vi "2D_array_statistics.vi"(4 "N Sig hist range":dbl=5.0 format="%.1f", 6 "Array":dbl[][](array[numeric])=array100x100[10000 elements] format="%.2f") -> (0 "1D array":dbl[](array[numeric]), 1 "mean 2":dbl=0.456875 format="%.2f", 2 "RMS 2":dbl=6.561297508877341 format="%.2f", 3 "median 3":dbl format="%.2f")   [LabVIEW 2017]
uses:
  <vilib>/Analysis/6fits.llb/Curve Fitting Criteria.ctl
  <vilib>/Analysis/5stat.llb/RMS (DBL).vi
  <vilib>/Analysis/baseanly.llb/Mean (DBL).vi
  <vilib>/Analysis/NI_AALBase.lvlib
  <vilib>/Analysis/NI_AALPro.lvlib
panel:
  out "RMS 2":dbl=6.561297508877341 format="%.2f"
  out "mean 2":dbl=0.456875 format="%.2f"
  out "median 2":dbl format="%.2f"
  out "Waveform Graph":dbl[](graph)
  in  "min":dbl=-45.47220756214139 format="%0.2f"
  in  "max":dbl=46.385957562141385 format="%0.2f"
  in  "# bins":i32=13
  out "# outside":cluster{"total":i32, "below":i32, "above":i32}={"total"=35, "below"=22, "above"=13}
  out "Histogram Graph":T1(graph)=[{"X Values"=[-41.93920121120744, -34.873188509339535, -27.80717580747163, -20.74116310560372, -13.675150403735815, -6.609137701867908, 0.4568749999999966, 7.5228877018679015, 14.588900403735806, 21.654913105603715, 28.720925807471623, 35.78693850933953, 42.85295121120743], "Histogram: h(x)"=[0, 0, 0, 17, 301, 1746, 3308, 2047, 414, 27, 1, 0, 0]}, {"X Values"=[-41.93920121120744, -34.873188509339535, -27.80717580747163, -20.74116310560372, -13.675150403735815, -6.609137701867908, 0.4568749999999966, 7.5228877018679015, 14.588900403735806, 21.654913105603715, 28.720925807471623, 35.78693850933953, 42.85295121120743], "Histogram: h(x)"=[16, 41, 106, 338, 911, 1746, 3317, 2047, 901, 377, 105, 44, 16]}]
  in  "method":T2=1 items=["Least Square", "Least Absolute Residual", "Bisquare"]
  out "Amplitude":dbl=3317.070983574361 format="%.2f"
  out "STDev":dbl=6.680329359755373 format="%.2f"
  out "Center":dbl=0.958994388159082 format="%.2f"
  out "auze 3":u32=10000
  out "auze 2":u32=2000
  out "auze":u32=8000
  out "size":u16[](array[numeric])=[100, 100]
  out "RMS":dbl=11.6418383428048 format="%.3g"
  out "mean":dbl=0.4562 format="%.3g"
  out "median":dbl format="%.3f"
  # "Least Absolute Residual"
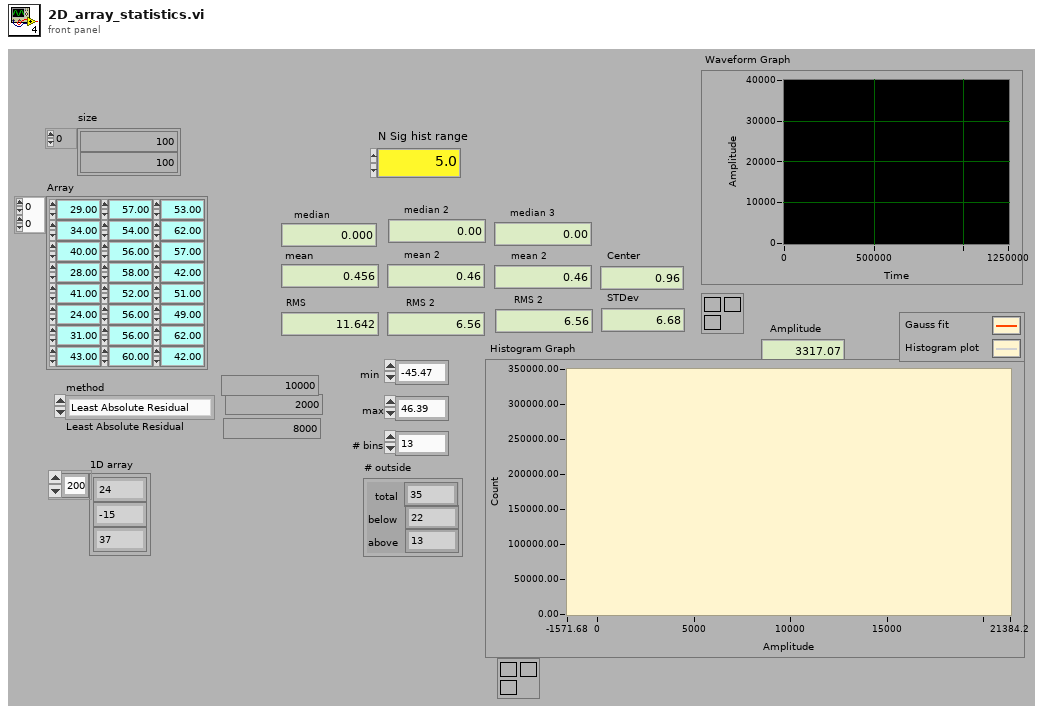
[diagram p1: front panel]
types:
  T1 = cluster{"X Values":dbl[], "Histogram: h(x)":i32[]}[]
  T2 = typedef "NI_AALPro.lvlib/Curve Fitting Criteria.ctl" = u16
  T3 = cluster{"X Values":dbl[], "Histogram: h(x)":i32[]}
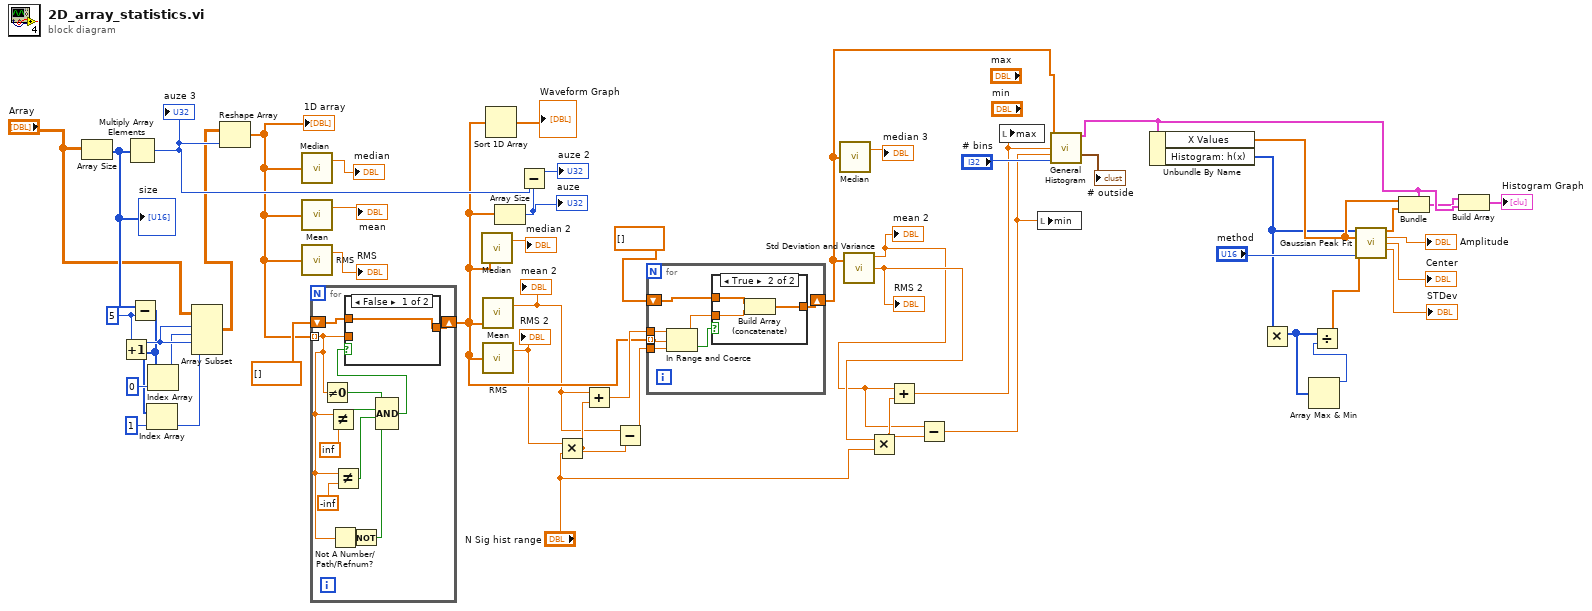
[diagram p0: block diagram]
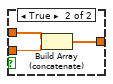
[diagram p3: hidden frame]
diagram:
  w29 = 5 ("y")
  n1 = Array Size(array="Array") -> (size(s)=w31:i32[])
  "size" <- w31
  n2 = Increment(x=w29) -> (x+1=w28:i32)
  n3 = Multiply Array Elements(1:w31) -> (0:w47:i32)
  "auze 3" <- w47
  n4 = Subtract(x=w31, y=w29) -> (x-y=w23:i32[])
  n5 = Index Array(array=w23, index=1) -> (element=w22:i32)
  n6 = Index Array(array=w23, index=0) -> (element=w25:i32)
  n7 = Array Subset(array="Array", index (row)=w28, length (row)=w25, index (col)=w28, length (col)=w22) -> (w24:dbl[][])
  n8 = Reshape Array(w24, w47) -> (w16:dbl[])
  "1D array" <- w16
  n9 = call <vilib>:"Median.vi"("X"=w16) -> ("median"=→"median":dbl)  [unwired: 1 out]
  n10 = call-poly <vilib>:"Mean.vi"("X"=w16) -> ("mean"=→"mean":dbl)  [unwired: 1 out]
  n11 = call-poly <vilib>:"RMS.vi"("X"=w16) -> ("rms value"=→"RMS":dbl)  [unwired: 1 out]
  n12 = for {
    tunnel: w16 -> [w53] mode=indexing
    shift-right: [w60] -> w7
    shift-left: dbl[] [] -> [w61]
    n13 = Not Equal To 0?(x=w53) -> (x != 0?=w57:bool)
    n14 = Not Equal?(x=w53, y=inf) -> (x != y?=w56:bool)
    n15 = Not A Number/Path/Refnum?(number/path/refnum=w53) -> (NaN/Path/Refnum?=w52:bool)
    n16 = Not Equal?(x=w53, y=-inf) -> (x != y?=w55:bool)
    n17 = Not(x=w52) -> (.not. x?=w51:bool)
    n18 = Compound Arithmetic op=AND(w57, w56, w55, w51) -> (w58:bool)
    n19 = case shown="False" w58 {
      tunnel: w53 -> [_ w65]
      tunnel: w61 -> [w62 w64]
      tunnel: [w62 w63] -> w60
      frame False {
      }
      frame True {
        n20 = Build Array (concatenate)(w64, w65) -> (w63:dbl[])
      }
    }
  }
  n21 = call <vilib>:"Median.vi"("X"=w7) -> ("median"=→"median 2":dbl)  [unwired: 1 out]
  n22 = call-poly <vilib>:"Mean.vi"("X"=w7) -> ("mean"=w3:dbl)  [unwired: 1 out]
  "mean 2" <- w3
  n23 = call-poly <vilib>:"RMS.vi"("X"=w7) -> ("rms value"=w4:dbl)  [unwired: 1 out]
  "RMS 2" <- w4
  n24 = Sort 1D Array(array=w7) -> (sorted array=→"Waveform Graph":dbl[])
  n25 = Array Size(array=w7) -> (size(s)=w49:i32)
  "auze" <- w49
  n26 = Subtract(x=w47, y=w49) -> (x-y=→"auze 2":i32)
  n27 = Multiply(x=w4, y="N Sig hist range") -> (x*y=w15:dbl)
  n28 = Add(x=w3, y=w15) -> (x+y=w11:dbl)
  n29 = Subtract(x=w3, y=w15) -> (x-y=w10:dbl)
  n30 = for {
    shift-right: [w71] -> w8
    shift-left: dbl[] [] -> [w72]
    tunnel: w7 -> [w70] mode=indexing
    tunnel: w11 -> [w69]
    tunnel: w10 -> [w68]
    n31 = In Range and Coerce(upper limit=w69, x=w70, lower limit=w68) -> (coerced(x)=w66:dbl, In Range?=w67:bool)
    n32 = case shown="True" w67 {
      tunnel: w66 -> [_ w76]
      tunnel: w72 -> [w73 w75]
      tunnel: [w73 w74] -> w71
      frame False {
      }
      frame True {
        n33 = Build Array (concatenate)(w75, w76) -> (w74:dbl[])
      }
    }
  }
  n34 = call <vilib>:"Median.vi"("X"=w8) -> ("median"=→"median 3":dbl)  [unwired: 1 out]
  n35 = call <vilib>:"Std Deviation and Variance.vi"("X"=w8) -> ("mean"=w1:dbl, "standard deviation"=w2:dbl)  [unwired: 1 in, 1 out]
  "mean 2" <- w1
  "RMS 2" <- w2
  n36 = Multiply(x=w2, y="N Sig hist range") -> (x*y=w32:dbl)
  n37 = Add(x=w1, y=w32) -> (x+y=w19:dbl)
  n38 = Subtract(x=w1, y=w32) -> (x-y=w20:dbl)
  n39 = local write "max"(w19) -> ()
  n40 = local write "min"(w20) -> ()
  n41 = call <vilib>:"General Histogram.vi"("X"=w8, "max"=w19, "min"=w20, "# bins"="# bins") -> ("Histogram Graph"=w40:T3, "# outside"=→"# outside":cluster{"total":i32, "below":i32, "above":i32})  [unwired: 7 in, 3 out]
  n42 = Unbundle By Name(w40) -> ("X Values"=w44:dbl[], "Histogram: h(x)"=w34:i32[])
  n43 = Multiply(x=w34, y=w34) -> (x*y=w36:i32[])
  n44 = Array Max & Min(array=w36) -> (max value=w43:i32)  [unwired: 3 out]
  n45 = Divide(x=w36, y=w43) -> (x/y=w35:dbl[])
  n46 = call <vilib>:"Gaussian Peak Fit.vi"("Y"=w34, "X"=w44, "Weight"=w35, "method"="method") -> ("Best Gaussian Fit"=w41:dbl[], "amplitude"=→"Amplitude":dbl, "center"=→"Center":dbl, "standard deviation"=→"STDev":dbl)  [unwired: 5 in, 3 out]
  n47 = Bundle(cluster=w40, "X Values"=w44, "Histogram: h(x)"=w41) -> (w39:T3)
  n48 = Build Array(w39, w40) -> (→"Histogram Graph":T1)
